vi "Add Parent UID To Child Node.vi"(7 "Replace? (F)":bool, 8 "error in (no error)":errorcluster, 9 "Child UID":string, 10 "Parent UID":string, 11 "Base Tree in":refnum<class "Base Tree.lvclass">) -> (0 "error out":errorcluster, 1 "Replaced?":bool, 3 "Base Tree out":refnum<class "Base Tree.lvclass">)   [LabVIEW 2017, in "opcua.lvlib" / "Browser Core.lvlib" / "Base Tree.lvclass"]
doc: "Add Parent UID to private data of Child Class with input UID.\n\nReplaced? output will return true if the Parent UID private data has been updated (Replace? input is TRUE and value is overwritten or if UID was empty and value was udpated)."
uses:
  Base Tree.lvclass
  Base Tree.lvclass/Base Tree.ctl
  Node Classes/Generic Node/Generic Node.lvclass
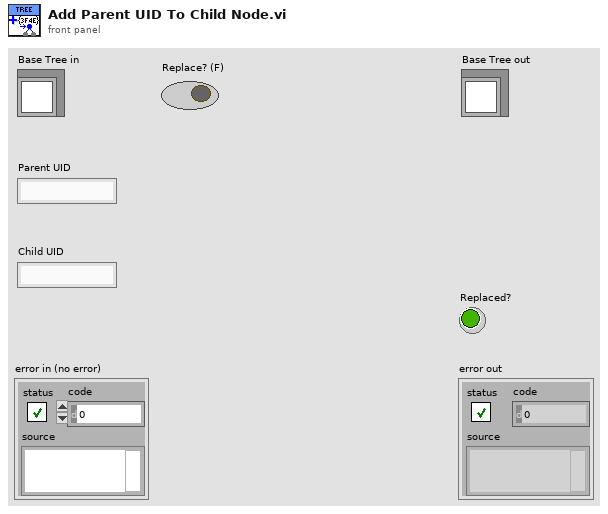
[diagram p1: front panel]
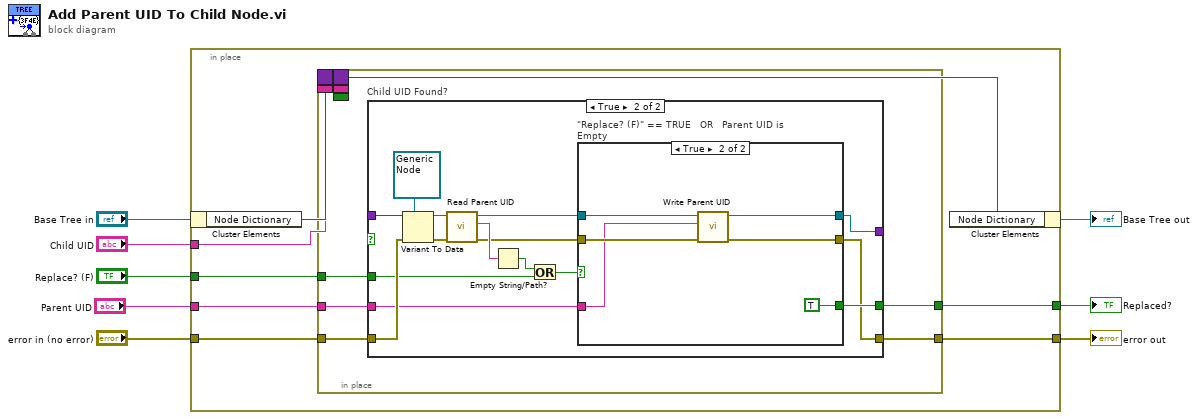
[diagram p0: block diagram]
diagram:
  n1 = in-place {
    in-place-border: "Child UID" -> [w15]
    in-place-border: "error in (no error)" -> [w14]
    in-place-border: "Replace? (F)" -> [w13]
    in-place-border: "Parent UID" -> [w12]
    in-place-border: [w11] -> w3
    in-place-border: [w10] -> w2
    n2 = in-place-cluster #1("Base Tree in") -> ("Node Dictionary"=w16:variant)
    n3 = in-place {
      border: w16 -> [_]
      border: w15 -> [_]
      border: [_] -> w9
      border: _ -> [_]
      border: _ -> [_]
      in-place-border: w14 -> [w22]
      in-place-border: w13 -> [w21]
      in-place-border: w12 -> [w20]
      in-place-border: [w19] -> w11
      in-place-border: [w18] -> w10
      n4 = case "Child UID Found?" shown="True" w24 {
        tunnel: w23 -> [w26 w41]
        tunnel: w22 -> [w25 w40]
        tunnel: w21 -> [_ w34]
        tunnel: w20 -> [_ w30]
        tunnel: [_ w29] -> w19
        tunnel: [w25 w28] -> w18
        tunnel: [w26 w27] -> w17
        frame False {
        }
        frame True {
          n5 = Variant To Data(error in=w40, type=refnum<class "Generic Node.lvclass"> refnum ("Browser Core.lvlib:Generic Node.lvclass"), Variant=w41) -> (data=w38:refnum<class "Generic Node.lvclass">, error out=w37:errorcluster)
          n6 = call "Read Parent UID.vi"("error in (no error)"=w37, "Generic Node in"=w38) -> ("error out"=w31:errorcluster, "Parent UID"=w36:string, "Generic Node out"=w32:refnum<class "Generic Node.lvclass">)  [unwired: 7 in]
          n7 = Empty String/Path?(string/path=w36) -> (empty?=w35:bool)
          n8 = Or(x=w35, y=w34) -> (x .or. y?=w33:bool)
          n9 = case "\"Replace? (F)\" == TRUE   OR   Parent UID is Empty" shown="True" w33 {
            tunnel: w32 -> [w43 w49]
            tunnel: w31 -> [w42 w48]
            tunnel: w30 -> [_ w47]
            tunnel: [_ TRUE] -> w29
            tunnel: [w43 w45] -> w27
            tunnel: [w42 w44] -> w28
            frame False {
              # "Do Not Replace Parent UID"
            }
            frame True {
              n10 = call "Write Parent UID.vi"("error in (no error)"=w48, "Parent UID"=w47, "Generic Node in"=w49) -> ("error out"=w44:errorcluster, "Generic Node out"=w45:refnum<class "Generic Node.lvclass">)  [unwired: 7 in]
            }
          }
        }
      }
    }
    n11 = in-place-cluster #1("Node Dictionary"=w9) -> (→"Base Tree out":refnum<class "Base Tree.lvclass">)
  }
  "error out" <- w2
  "Replaced?" <- w3
